vi "PIC2_DEMO.vi"() -> ()   [LabVIEW 2016]
uses:
  <vilib>/picture/picture.llb/Draw True-Color Pixmap.vi
panel:
  out "R":u8
  in  "Color Box":u32(colorbox)=16860
  out "B":u8
  out "G":u8
  out "new picture 2":picture
  out "new picture":picture
  in  "# OF COLUMNS":i32
  in  "# OF ROWS":i32
  in  "top left point(0, 0)":cluster{"x":i16, "y":i16}
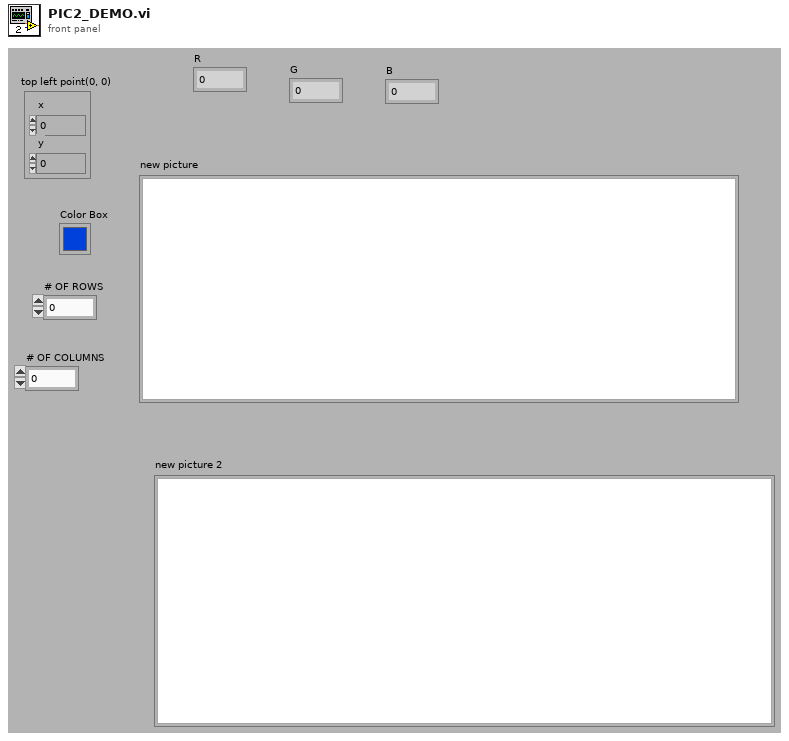
[diagram p1: front panel]
types:
  T1 = typedef "imagedata.ctl" = cluster{"image type":i32, "image depth":i32, "image":u8[], "mask":u8[], "colors":u32[], "Rectangle":cluster{"left":i16, "top":i16, "right":i16, "bottom":i16}}
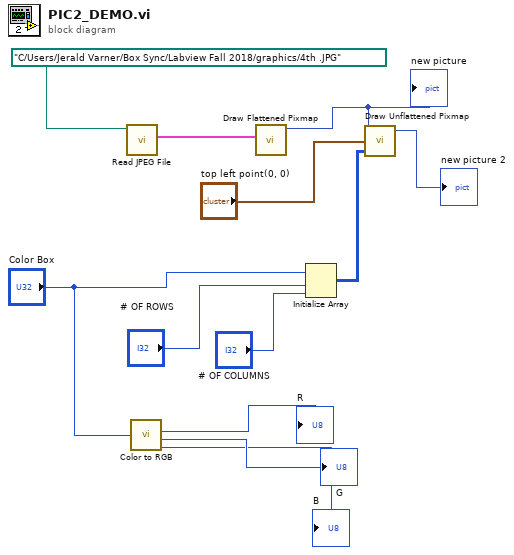
[diagram p0: block diagram]
diagram:
  n1 = call <vilib>:"Read JPEG File.vi"("path to JPEG file"=path "C:/Users/Jerald Varner/Box Sync/Labview Fall 2018/graphics/4th .JPG") -> ("image data"=w12:T1)  [unwired: 8 in, 2 out]
  n2 = call <vilib>:"Color to RGB.vi"("Color"="Color Box") -> ("R"=→"R":u8, "G"=→"G":u8, "B"=→"B":u8)  [unwired: 1 out]
  n3 = call <vilib>:"Draw Flattened Pixmap.vi"("image data"=w12) -> ("new picture"=w11:picture)  [unwired: 8 in]
  "new picture" <- w11
  n4 = Initialize Array "Initialize Array"("Color Box", "# OF ROWS", "# OF COLUMNS") -> (w7:u32[][])
  n5 = call-poly <vilib>:"Draw Unflattened Pixmap.vi"("picture"=w11, "top left point(0, 0)"="top left point(0, 0)", "data (RGB format)"=w7) -> ("new picture"=→"new picture 2":picture)  [unwired: 6 in]
